vi "Get Size of Data from TD - Variant String - Returns Correct Size.vi"() -> ()   [LabVIEW 2017, in "Composition.Tests.lvlib"]
uses:
  Composition.Tests.lvlib
  <vilib>/addons/_JKI Toolkits/Caraya/classes/Assert/Assert Equal Value_Variant.vi
  Composition/Composition.lvlib
  <vilib>/addons/_JKI Toolkits/Caraya/classes/Test/Test.lvclass
  <vilib>/addons/_JKI Toolkits/Caraya/classes/Assert/Assert.lvclass
panel:
  out "error out":errorcluster
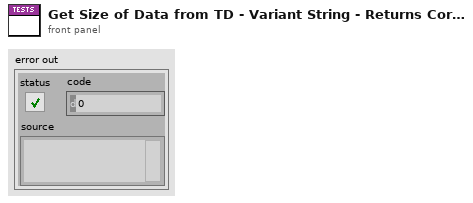
[diagram p1: front panel]
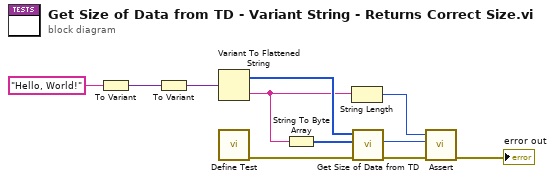
[diagram p0: block diagram]
diagram:
  n1 = To Variant(anything="Hello, World!") -> (Variant=w10:variant)
  n2 = To Variant(anything=w10) -> (Variant=w7:variant)
  n3 = Variant To Flattened String(Variant=w7) -> (data string=w2:string, 1:w9:i16[])
  n4 = call <vilib>:"Define Test.vi"() -> ("error out"=w6:errorcluster)  [unwired: 10 in, 1 out]
  n5 = String To Byte Array(string=w2) -> (unsigned byte array=w8:u8[])
  n6 = String Length(string=w2) -> (length=w1:i32)
  n7 = call "Get Size of Data from TD.vi"("error in (no error)"=w6, "Data String"=w8, "Type Descriptor"=w9) -> ("error out"=w5:errorcluster, "Size of Data"=w4:i32)  [unwired: 7 in]
  n8 = call-poly <vilib>:"Assert.vi"("error in (no error)"=w5, "Y"=w4, "X"=w1) -> ("error out"=→"error out":errorcluster)  [unwired: 7 in, 1 out]
